vi "Pump Refill.vi"(6 "auto_switch_valve":bool=TRUE, 8 "error in (no error)":errorcluster, 9 "Refill flow rate, uL/s":dbl=200.0, 11 "Application in":refnum<class "Application.lvclass">) -> (0 "error out":errorcluster, 3 "Application out":refnum<class "Application.lvclass">)   [LabVIEW 2018, in "Application.lvlib" / "Application.lvclass"]
uses:
  Application.lvclass
  Application.lvclass/Application.ctl
  Hardware/PHD Ultra Messages/Run Withdraw Msg/Run Refill Msg.lvclass/Run Refill Msg.ctl
  <vilib>/ActorFramework/Message Enqueuer/Message Enqueuer.lvclass/Message Enqueuer.ctl
  <vilib>/ActorFramework/Message Enqueuer/Enqueue.vi
  Hardware/PHD Ultra Messages/Run Withdraw Msg/Run Refill Msg.lvclass
  C:/Program Files/National Instruments/LabVIEW 2018/vi.lib/ActorFramework/Message/Message.lvclass
  <vilib>/ActorFramework/Message Priority Queue/Priority Enqueue.vi
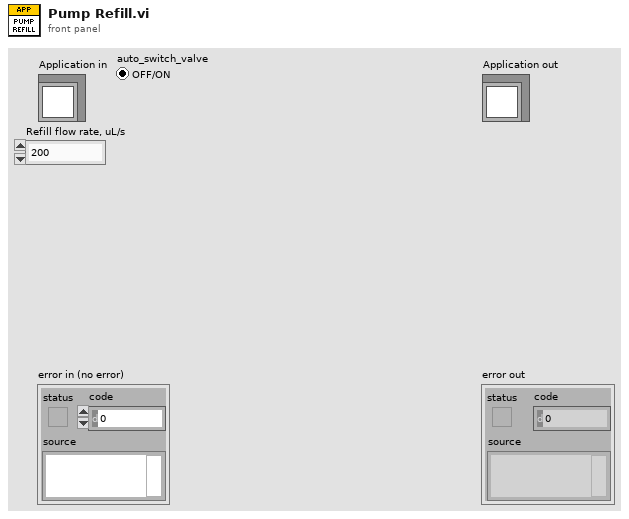
[diagram p1: front panel]
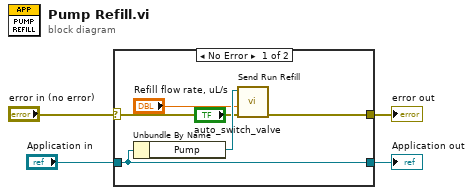
[diagram p0: block diagram]
diagram:
  n1 = case shown="No Error" "error in (no error)" {
    selector: "error in (no error)" -> [w8 w12]
    tunnel: [w7 w12] -> w3
    tunnel: [w10 w11] -> w1
    tunnel: "Application in" -> [w10 w11]
    frame No Error {
      n2 = Unbundle By Name(w10) -> ("Pump"=w9:refnum<class "Message Enqueuer.lvclass">)
      n3 = call "Send Run Refill.vi"("auto_switch_valve"="auto_switch_valve", "error in (no error)"=w8, "Refill flow rate, uL/s"="Refill flow rate, uL/s", "Message Enqueuer"=w9) -> ("error out"=w7:errorcluster)  [unwired: 6 in, 1 out]
    }
    frame Error {
    }
  }
  "error out" <- w3
  "Application out" <- w1
